vi "RT Host - calc perp dist from des traj.vi"(7 "Current Global W/S Pos (mm)":dbl[](array[numeric])=[0.0, -90.0], 8 "error in (no error)":errorcluster, 10 "Yint Global W/S (mm)":dbl, 11 "Xint Global W/S (mm)":dbl) -> (0 "error out":errorcluster, 3 "Perp Dist Global W/S (mm)":dbl)   [LabVIEW 2017]
doc: "This subVI calculates the perpendicular distance of the current position from the desired trajectory."
panel:
  # "Inputs"
  # "Outputs"
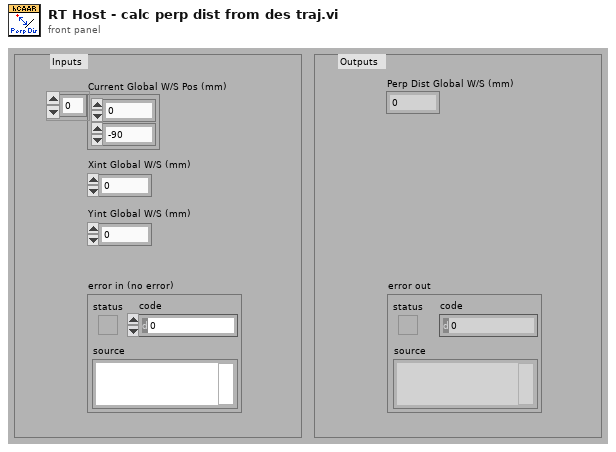
[diagram p1: front panel]
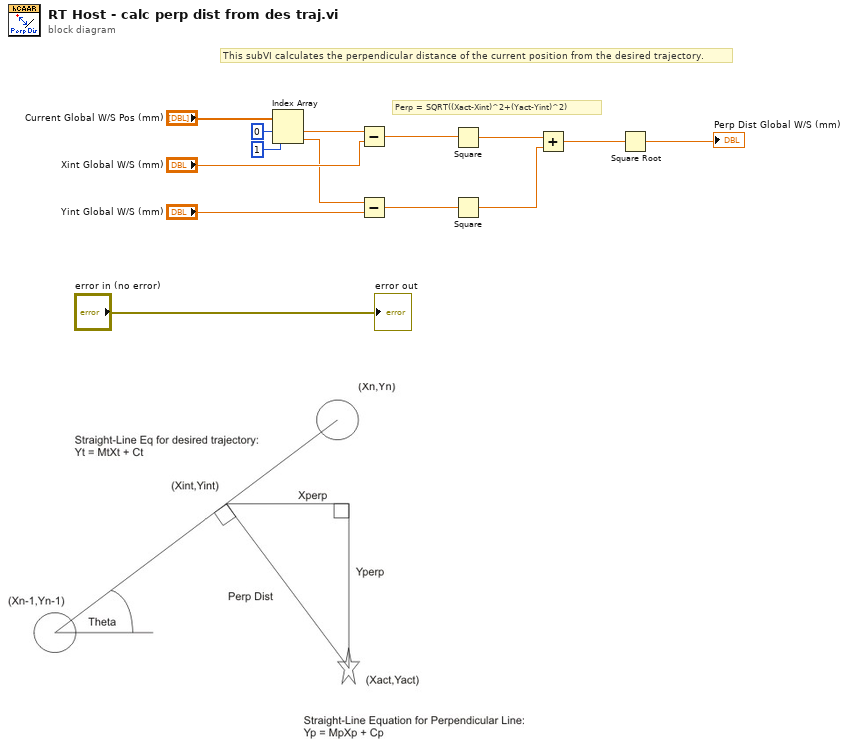
[diagram p0: block diagram]
diagram:
  # "Perp = SQRT((Xact-Xint)^2+(Yact-Yint)^2)"
  # "This subVI calculates the perpendicular distance of the current position from the desired trajectory."
  n1 = Index Array(array="Current Global W/S Pos (mm)", index #1=0 ("index"), index #2=1 ("index")) -> (element #1=w10:dbl, element #2=w7:dbl)
  n2 = Subtract(x=w10, y="Xint Global W/S (mm)") -> (x-y=w6:dbl)
  n3 = Subtract(x=w7, y="Yint Global W/S (mm)") -> (x-y=w5:dbl)
  n4 = Square(x=w6) -> (x^2=w4:dbl)
  n5 = Square(x=w5) -> (x^2=w3:dbl)
  n6 = Add(x=w4, y=w3) -> (x+y=w2:dbl)
  n7 = Square Root(x=w2) -> (sqrt(x)=→"Perp Dist Global W/S (mm)":dbl)
  "error out" <- "error in (no error)"
